vi "TimeoutSkill.vi"(6 "IndexInVector":dbl, 8 "error in (no error)":errorcluster, 9 "Game":refnum<class "Game.lvclass">, 10 "Robot":refnum<class "Robot.lvclass">, 11 "TimeoutSkill in":refnum<class "TimeoutSkill.lvclass">) -> (0 "error out":errorcluster, 2 "Robot out":refnum<class "Robot.lvclass">, 3 "TimeoutSkill out":refnum<class "TimeoutSkill.lvclass">)   [LabVIEW 2018, in "TimeoutSkill.lvclass"]
uses:
  TimeoutSkill.lvclass
  Robot_class/Robot.lvclass
  Game_class/Game.lvclass
  Game_class/Game.lvclass/Game.ctl
  Parameters_class/Parameters.lvclass/Parameters.ctl
  Robot_class/Robot.lvclass/Robot.ctl
  Game_class/Read FieldRef.vi
  Game_class/Read Parameters.lvclass.vi
  Parameters_class/Read TimeoutDistanceBetweenRobots.vi
  Parameters_class/Read TimeoutDistanceInX.vi
  Parameters_class/Read TimeoutDistanceInY.vi
  Robot_class/Write dest_x.vi
  Robot_class/Write dest_y.vi
  Robot_class/Write dest_orientation.vi
  Field_class/Field.lvclass
  Parameters_class/Parameters.lvclass
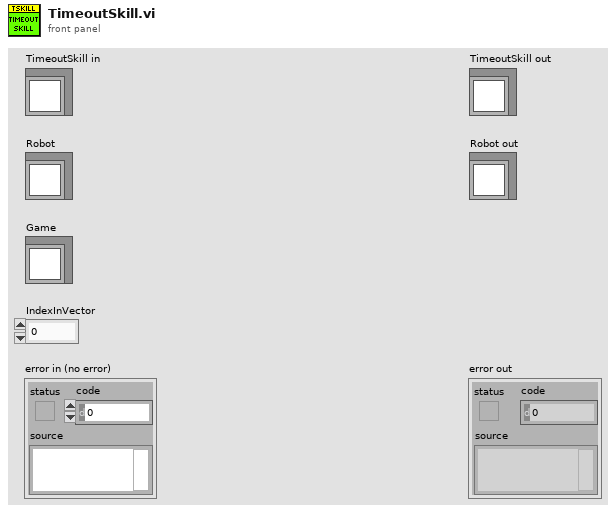
[diagram p1: front panel]
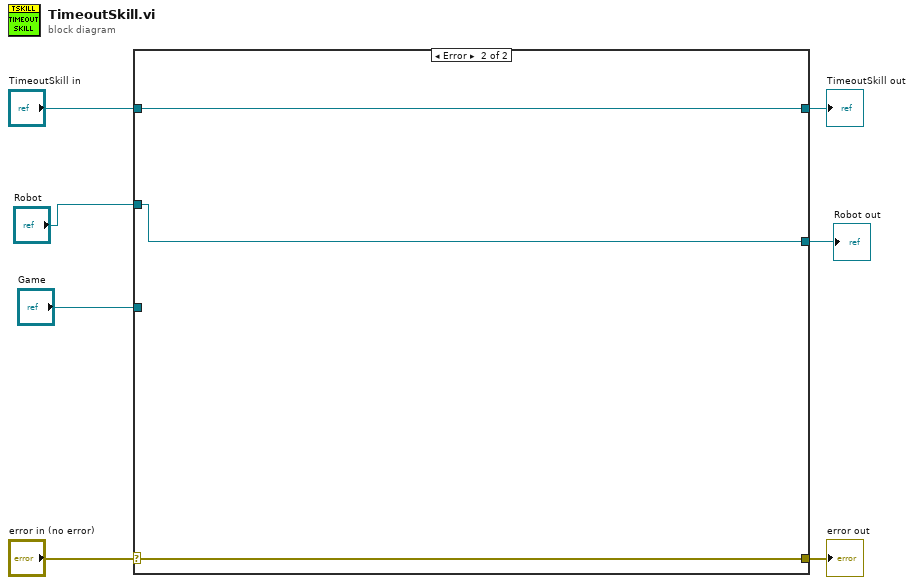
[diagram p0: block diagram]
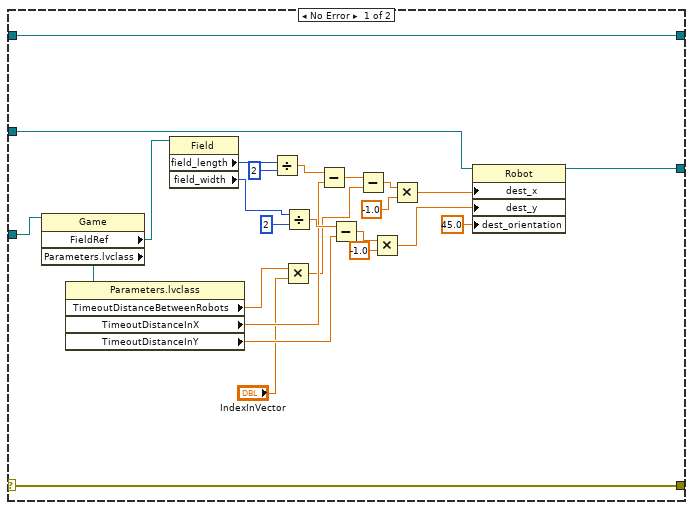
[diagram p2: hidden frame]
diagram:
  n1 = case shown="Error" "error in (no error)" {
    selector: "error in (no error)" -> [w32 w36]
    tunnel: [w32 w36] -> w6
    tunnel: [w33 w35] -> w4
    tunnel: "TimeoutSkill in" -> [w33 w35]
    tunnel: "Game" -> [w31 _]
    tunnel: "Robot" -> [w12 w34]
    tunnel: [w8 w34] -> w1
    frame No Error {
      n2 = property class="Game"(reference=w31) -> ("FieldRef"=w29:refnum<class "Field.lvclass">, "Parameters.lvclass"=w30:refnum<class "Parameters.lvclass">)  [unwired: 1 in, 2 out]
      n3 = property class="Parameters.lvclass"(reference=w30) -> ("TimeoutDistanceBetweenRobots"=w18:dbl, "TimeoutDistanceInX"=w20:dbl, "TimeoutDistanceInY"=w22:dbl)  [unwired: 1 in, 2 out]
      n4 = property class="Field"(reference=w29) -> ("field_length"=w28:i32, "field_width"=w23:i32)  [unwired: 1 in, 2 out]
      n5 = Divide(x=w28, y=2) -> (x/y=w21:dbl)
      n6 = Multiply(x=w18, y="IndexInVector") -> (x*y=w16:dbl)
      n7 = Divide(x=w23, y=2) -> (x/y=w25:dbl)
      n8 = Subtract(x=w21, y=w20) -> (x-y=w19:dbl)
      n9 = Subtract(x=w25, y=w22) -> (x-y=w24:dbl)
      n10 = Subtract(x=w19, y=w16) -> (x-y=w14:dbl)
      n11 = Multiply(x=w24, y=-1.0) -> (x*y=w10:dbl)
      n12 = Multiply(x=w14, y=-1.0) -> (x*y=w11:dbl)
      n13 = property class="Robot"(reference=w12, "dest_x"=w11, "dest_y"=w10, "dest_orientation"=45.0) -> (reference out=w8:refnum<class "Robot.lvclass">)  [unwired: 1 in, 1 out]
    }
    frame Error {
    }
  }
  "error out" <- w6
  "TimeoutSkill out" <- w4
  "Robot out" <- w1
